vi "求水仙花数.vi"(1 "结束数":i32=999, 2 "开始数":i32=100) -> (0 "水仙花数":i32[](array[numeric]))   [LabVIEW 2012]
doc: "功能：\n\n求三位数中的水仙花数\n\n水仙花数的定义：\n\n所谓水仙花数，是指一个三位数，其各个位数的立方和等于该数本身，比如：\n\n153=1^3+5^+3^\n\ncsxcs_366创建"
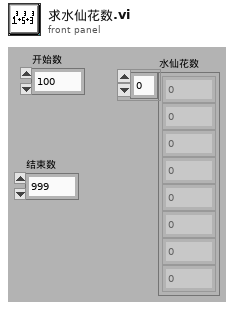
[diagram p1: front panel]
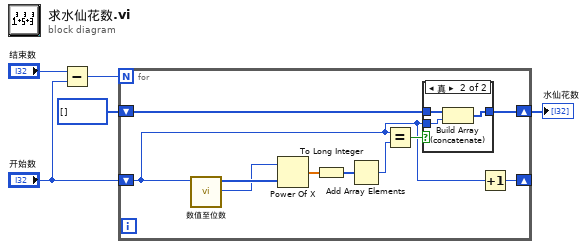
[diagram p0: block diagram]
diagram:
  n1 = Subtract(x="结束数", y="开始数") -> (x-y=w5:i32)
  n2 = for {
    N: w5 -> [_]
    shift-right: [w12] -> _
    shift-left: "开始数" -> [w13]
    shift-right: [w10] -> w3
    shift-left: i32[] [] -> [w11]
    n3 = call-poly "数值至位数.vi"("输入数值"=w13) -> ("总位数"=w6:i32, "位数数组"=w7:i32[])  [unwired: 8 in, 1 out]
    n4 = Power Of X(1:w7, 2:w6) -> (0:w9:dbl[])
    n5 = To Long Integer(number=w9) -> (32bit integer=w8:i32[])
    n6 = Add Array Elements(numeric array=w8) -> (sum=w15:i32)
    n7 = Equal?(x=w13, y=w15) -> (x = y?=w14:bool)
    n8 = case shown="真" w14 {
      tunnel: w11 -> [w16 w17]
      tunnel: [w16 w18] -> w10
      tunnel: w13 -> [_ w19]
      frame False {
      }
      frame True {
        n9 = Build Array (concatenate)(w17, w19) -> (w18:i32[])
      }
    }
    n10 = Increment(x=w13) -> (x+1=w12:i32)
  }
  "水仙花数" <- w3
